vi "ServoCount.vi"(8 "error in (no error)":errorcluster, 11 "Device In":i32) -> (0 "error out":errorcluster, 2 "Count":i32, 3 "Device Out":i32)   [LabVIEW 2012]
uses:
  phidget21.dll
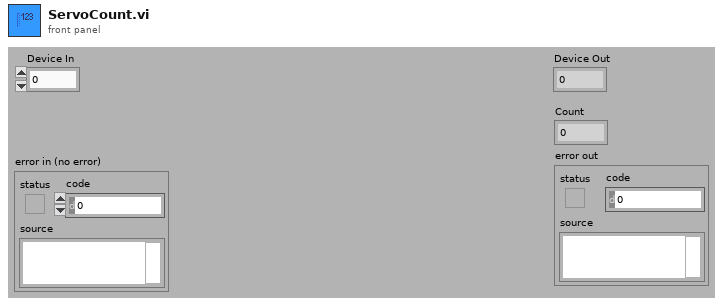
[diagram p1: front panel]
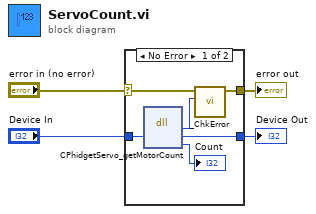
[diagram p0: block diagram]
diagram:
  n1 = case shown="No Error" "error in (no error)" {
    selector: "error in (no error)" -> [w8 w12]
    tunnel: [w7 w12] -> w3
    tunnel: "Device In" -> [w6 w11]
    tunnel: [w5 w11] -> w1
    frame No Error {
      n2 = dll-call lib="phidget21.*" fn="CPhidgetServo_getMotorCount"("phid"=w6) -> (w9:i32, "phid"=w5:i32, "count"=→"Count":i32)  [unwired: 4 in, 2 out]
      n3 = call "_ChkError.vi"("Return Code"=w9, "error in (no error)"=w8) -> ("error out"=w7:errorcluster)  [unwired: 9 in]
    }
    frame Error {
    }
  }
  "error out" <- w3
  "Device Out" <- w1
